vi "SLSC Update Values in Tree Control.vi"(0 "Section Ref in":T3 format="%.0x", 1 "TreeControl in":refnum<vi>, 2 "Properties":string="Properties", 3 "Command Channel":string="Commands", 5 "Property tree in":string[](array[string]), 7 "NewVal":variant, 9 "SLSC Output Tree":T1(array[cluster]), 11 "error in (no error)":errorcluster, 12 "Enums":T2[](array[typedef]), 13 "Enum Strings":cluster{"name":string, string}[](array[cluster]), 14 "Modify Reset Value?":bool) -> (10 "SLSC Output Tree Out":T1(array[cluster]), 15 "error out":errorcluster)   [LabVIEW 2015, in "SLSC EDS System Explorer.lvlib"]
uses:
  SLSC EDS System Explorer.lvlib
  <vilib>/NI Veristand/Custom Device API/Custom Device Item Ref.ctl
  SLSC EDS API/JSON parsing/enum.ctl
  <vilib>/NI Veristand/Custom Device Tools/Custom Device Utility Library/NI VeriStand - Search for Item by Name.vi
  SLSC UI API/SLSC Tree Control.lvlib
  <vilib>/NI VeriStand/Custom Device Tools/Custom Device Utility Library/Custom Device Utility Library.lvlib
  <vilib>/NI VeriStand/Custom Device API/Custom Device API.lvlib
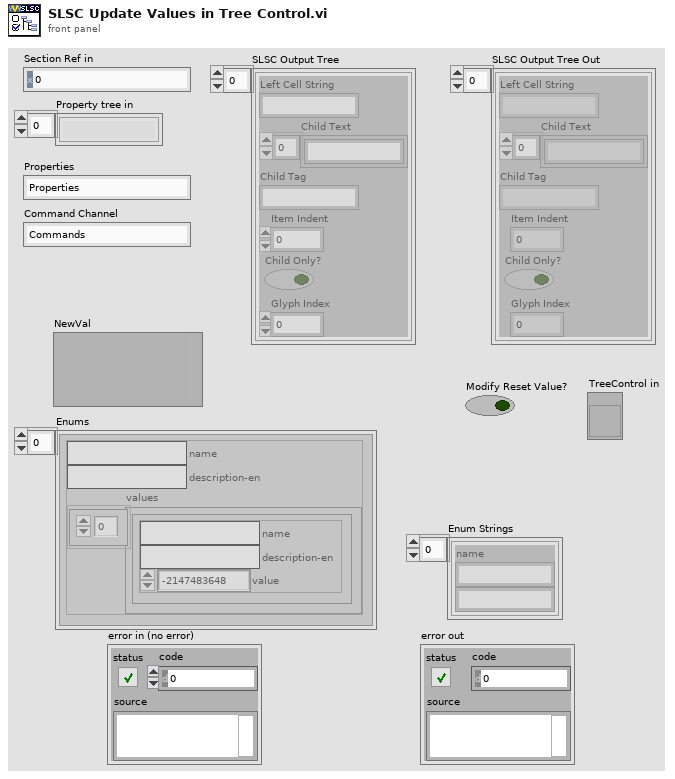
[diagram p1: front panel]
types:
  T1 = cluster{"Left Cell String":string, "Child Text":string[], "Child Tag":string, "Item Indent":i32, "Child Only?":bool, "Glyph Index":i32}[]
  T2 = typedef "enum.ctl" = cluster{"name":string, "description-en":string, "values":cluster{"name":string, "description-en":string, "value":i32}[]}
  T3 = typedef "Custom Device API.lvlib/Custom Device Item Ref.ctl" = u64
  T4 = cluster{"Left Cell String":string, "Child Text":string[], "Child Tag":string, "Item Indent":i32, "Child Only?":bool, "Glyph Index":i32}
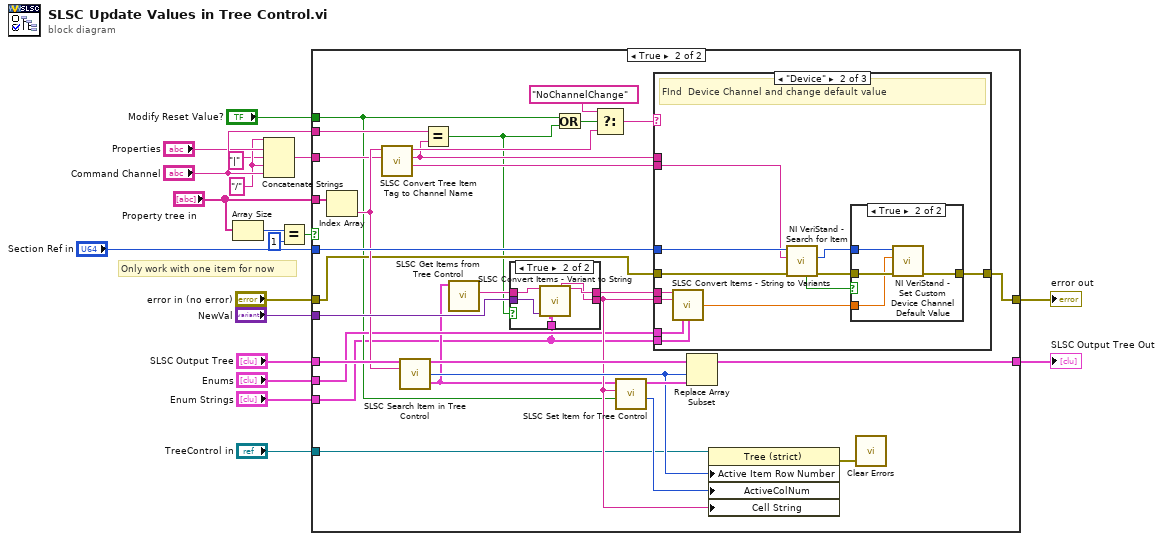
[diagram p0: block diagram]
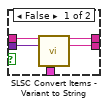
[diagram p3: hidden frame]
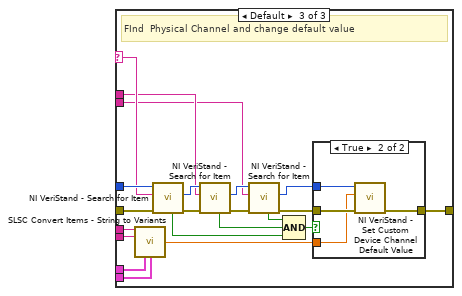
[diagram p6: hidden frame]
diagram:
  w14 = "/" ("string")
  # "Only work with one item for now"
  n1 = Array Size(array="Property tree in") -> (size(s)=w4:i32)
  n2 = Concatenate Strings(w14, "Properties", "|" ("string"), w14, "Command Channel") -> (w16:string)
  n3 = Equal?(x=w4, y=1) -> (x = y?=w3:bool)
  n4 = case shown="True" w3 {
    tunnel: "Section Ref in" -> [_ w44]
    tunnel: "SLSC Output Tree" -> [w21 w51]
    tunnel: "Enums" -> [_ w37]
    tunnel: "NewVal" -> [_ w46]
    tunnel: "Property tree in" -> [_ w50]
    tunnel: [w21 w47] -> w12
    tunnel: "Enum Strings" -> [_ w23]
    tunnel: "error in (no error)" -> [w20 w39]
    tunnel: [w20 w38] -> w11
    tunnel: w16 -> [_ w30]
    tunnel: "Command Channel" -> [_ w29]
    tunnel: "Modify Reset Value?" -> [_ w27]
    tunnel: "TreeControl in" -> [_ w26]
    frame False {
    }
    frame True {
      n5 = Index Array(array=w50) -> (element=w43:string)  [unwired: 1 in]
      n6 = call "SLSC Convert Tree Item Tag to Channel Name.vi"("Type of Item"=w30, "Item String"=w43) -> ("Item Name"=w42:string, "Type of Item"=w31:string, "Device/Physical Channel"=w32:string)  [unwired: 7 in]
      n7 = call "SLSC Search Item in Tree Control.vi"("SLSC Output Tree"=w51, "Item Tag"=w43) -> ("SLSC Output Tree Out"=w49:T1, "Position"=w45:i32, "Item"=w36:T4)  [unwired: 10 in, 1 out]
      n8 = Equal?(x=w29, y=w31) -> (x = y?=w22:bool)
      n9 = call "SLSC Get Items from Tree Control.vi"("Item"=w36) -> ("Datatype"=w24:string)  [unwired: 6 in, 4 out]
      n10 = case shown="True" w22 {
        tunnel: w46 -> [w56 w58]
        tunnel: [w55 w57] -> w41
        tunnel: [w54 w61] -> w40
        tunnel: w24 -> [w53 w60]
        tunnel: w23 -> [w52 w59]
        frame False {
          n11 = call "SLSC Convert Items - Variant to String.vi"("Datatype"=w53, "value"=w56, "Enum string"=w52) -> ("Output data type"=w54:string, "string data value"=w55:string)  [unwired: 6 in, 5 out]
        }
        frame True {
          n12 = call "SLSC Convert Items - Variant to String.vi"("Datatype"=w60, "reset value"=w58, "Enum string"=w59) -> ("string data reset value"=w57:string, "Output data type"=w61:string)  [unwired: 6 in, 5 out]
        }
      }
      n13 = Or(x=w27, y=w22) -> (x .or. y?=w28:bool)
      n14 = Select(t="NoChannelChange", s=w28, f=w32) -> (s? t:f=w35:string)
      n15 = call "SLSC Set Item for Tree Control.vi"("Modify Reset Value?"=w27, "Value"=w41, "Item In"=w36) -> ("Changed Column"=w33:i32, "Item Out"=w48:T4)  [unwired: 7 in]
      n16 = case shown="\"Device\"" w35 {
        selector: w35 -> [_ _ w97]
        tunnel: w44 -> [_ w74 w100]
        tunnel: w42 -> [_ w73 w90]
        tunnel: w41 -> [_ w66 w87]
        tunnel: w40 -> [_ w67 w88]
        tunnel: w39 -> [w62 w70 w99]
        tunnel: [w62 w68 w98] -> w38
        tunnel: w23 -> [_ w64 w85]
        tunnel: w37 -> [_ w65 w86]
        tunnel: w31 -> [_ _ w91]
        frame "NoChannelChange" {
          # "Do nothing"
        }
        frame "Device" {
          # "FInd  Device Channel and change default value"
          n17 = call "SLSC Convert Items - String to Variants.vi"("Datatype"=w67, "Value"=w66, "enums"=w65, "string enums"=w64) -> ("Value (DBL)"=w63:dbl)  [unwired: 8 in, 3 out]
          n18 = call-poly <vilib>:"NI VeriStand - Search for Item.vi"("error in"=w70, "Item Name"=w73, "Section Ref in"=w74) -> ("error out"=w69:errorcluster, "Item Ref"=w71:T3, "Found"=w72:bool)  [unwired: 5 in, 1 out]
          n19 = case shown="True" w72 {
            tunnel: w71 -> [_ w79]
            tunnel: w69 -> [w75 w78]
            tunnel: [w75 w77] -> w68
            tunnel: w63 -> [_ w76]
            frame False {
            }
            frame True {
              n20 = call <vilib>:"NI VeriStand - Set Custom Device Channel Default Value.vi"("error in (no error)"=w78, "Default Value"=w76, "Channel Ref in"=w79) -> ("error out"=w77:errorcluster)  [unwired: 7 in, 1 out]
            }
          }
        }
        frame Default {
          # "FInd  Physical Channel and change default value"
          n21 = call "SLSC Convert Items - String to Variants.vi"("Datatype"=w88, "Value"=w87, "enums"=w86, "string enums"=w85) -> ("Value (DBL)"=w84:dbl)  [unwired: 8 in, 3 out]
          n22 = call-poly <vilib>:"NI VeriStand - Search for Item.vi"("error in"=w99, "Item Name"=w97, "Section Ref in"=w100) -> ("error out"=w96:errorcluster, "Item Ref"=w95:T3, "Found"=w80:bool)  [unwired: 5 in, 1 out]
          n23 = call-poly <vilib>:"NI VeriStand - Search for Item.vi"("error in"=w96, "Item Name"=w91, "Section Ref in"=w95) -> ("error out"=w94:errorcluster, "Item Ref"=w93:T3, "Found"=w81:bool)  [unwired: 5 in, 1 out]
          n24 = call-poly <vilib>:"NI VeriStand - Search for Item.vi"("error in"=w94, "Item Name"=w90, "Section Ref in"=w93) -> ("error out"=w89:errorcluster, "Item Ref"=w92:T3, "Found"=w82:bool)  [unwired: 5 in, 1 out]
          n25 = Compound Arithmetic op=AND(w82, w81, w80) -> (w83:bool)
          n26 = case shown="True" w83 {
            tunnel: w92 -> [_ w105]
            tunnel: w89 -> [w101 w104]
            tunnel: [w101 w103] -> w98
            tunnel: w84 -> [_ w102]
            frame False {
            }
            frame True {
              n27 = call <vilib>:"NI VeriStand - Set Custom Device Channel Default Value.vi"("error in (no error)"=w104, "Default Value"=w102, "Channel Ref in"=w105) -> ("error out"=w103:errorcluster)  [unwired: 7 in, 1 out]
            }
          }
        }
      }
      n28 = Replace Array Subset(array=w49, new element=w48, index=w45) -> (w47:T1)
      n29 = property class="Tree (strict)"(reference=w26, "Active Item Row Number"=w45, "ActiveColNum"=w33, "Cell String"=w41) -> (error out=w25:errorcluster)  [unwired: 1 in, 1 out]
      n30 = call <vilib>:"Clear Errors.vi"("error in (no error)"=w25) -> ()  [unwired: 5 in, 2 out]
    }
  }
  "SLSC Output Tree Out" <- w12
  "error out" <- w11
